vi "Set Front Panel Visibility.vi"(6 "Set Value":bool, 9 "Elapsed Time":dbl, 10 "Current Tab":T1(ring), 11 "output cluster":T2) -> (3 "New Tab":T1(ring))   [LabVIEW 2016]
uses:
  Controls/Cal Refs.ctl
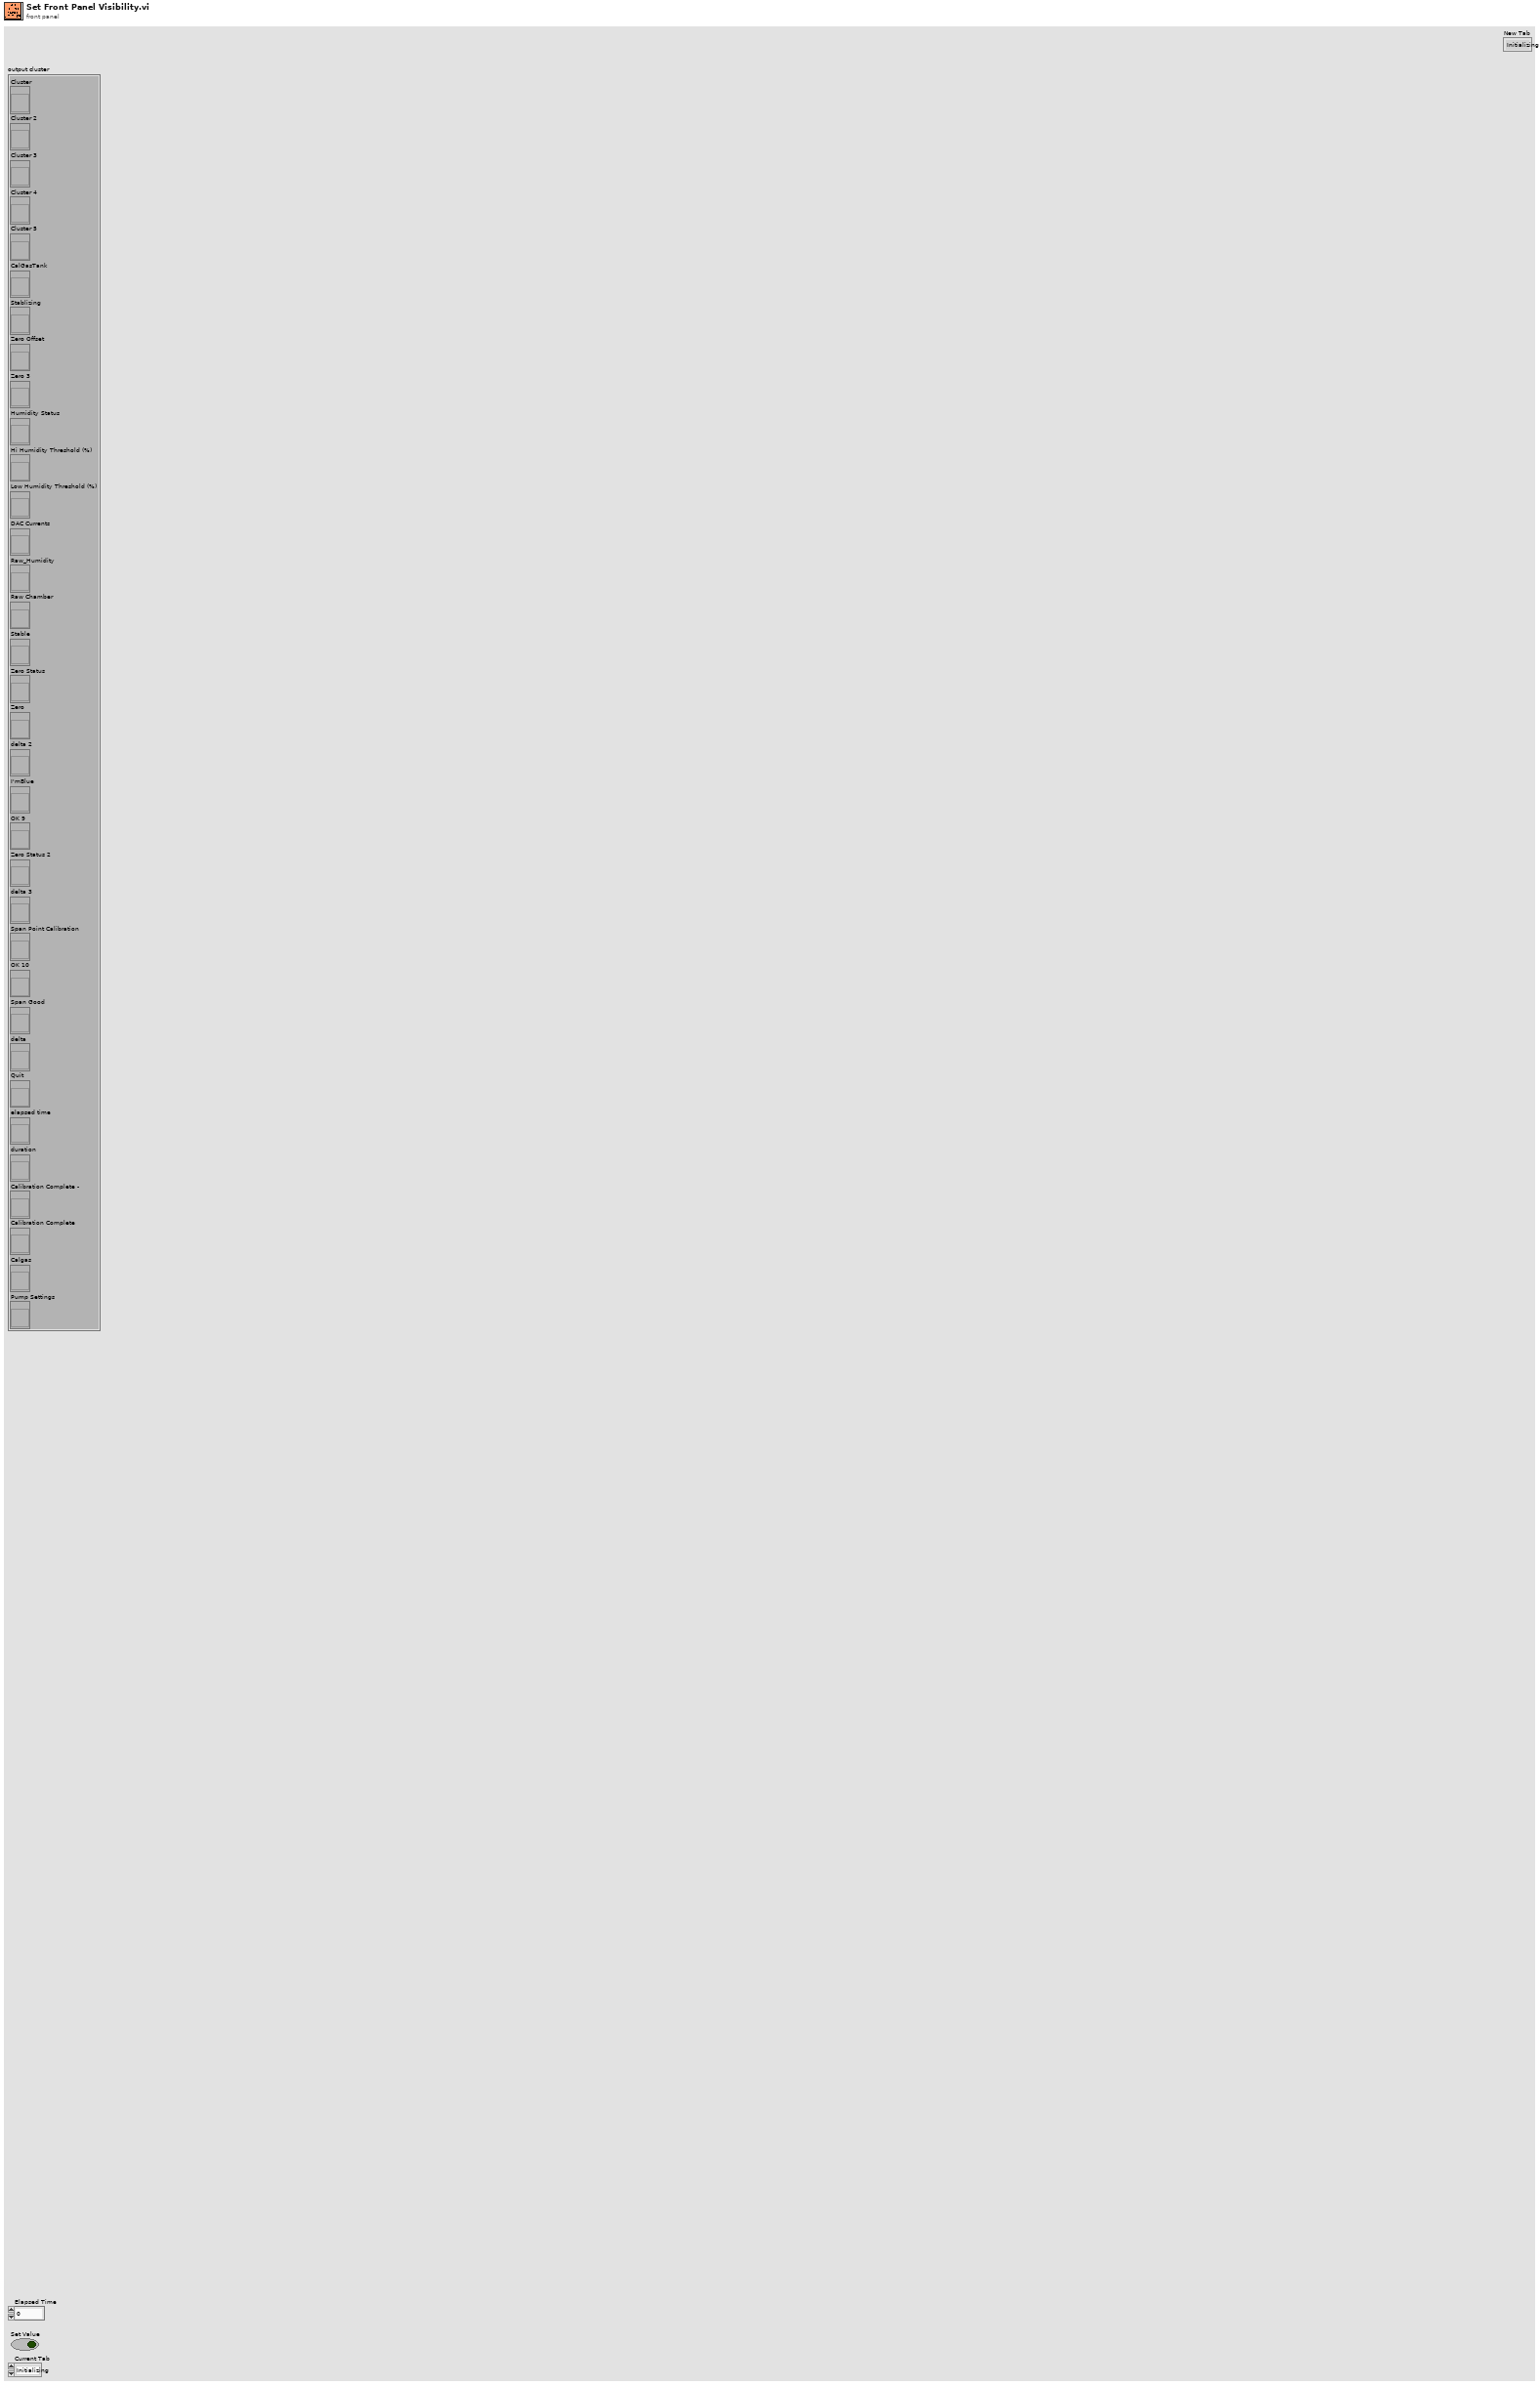
[diagram p1: front panel]
types:
  T1 = enum32{"Initializing", "Enter CO2 Value", "Enter Calibration Code", "Reading Calibration Data", "Stablizing", "Calculating Target Voltages", "Setting Zero Point", "Setting High Point", "Setting Span Point", "Calculating Gain & Offset", "Storing Calibration Coefficients", "Calibration Complete"}
  T2 = typedef "Cal Refs.ctl" = cluster{"Cluster":refnum<vi>, "Cluster 2":refnum<vi>, "Cluster 3":refnum<vi>, "Cluster 4":refnum<vi>, "Cluster 5":refnum<vi>, "CalGasTank":refnum<vi>, "Stablizing":refnum<vi>, "Zero Offset":refnum<vi>, "Zero 3":refnum<vi>, "Humidity Status":refnum<vi>, "Hi Humidity Threshold (%)":refnum<vi>, "Low Humidity Threshold (%)":refnum<vi>, "DAC Currents":refnum<vi>, "Raw_Humidity":refnum<vi>, "Raw Chamber":refnum<vi>, "Stable":refnum<vi>, "Zero Status":refnum<vi>, "Zero":refnum<vi>, "delta 2":refnum<vi>, "I'mBlue":refnum<vi>, "OK 9":refnum<vi>, "Zero Status 2":refnum<vi>, "delta 3":refnum<vi>, "Span Point Calibration":refnum<vi>, "OK 10":refnum<vi>, "Span Good":refnum<vi>, "delta":refnum<vi>, "Quit":refnum<vi>, "elapsed time":refnum<vi>, "duration":refnum<vi>, "Calibration Complete -":refnum<vi>, "Calibration Complete":refnum<vi>, "Calgas":refnum<vi>, "Pump Settings":refnum<vi>}
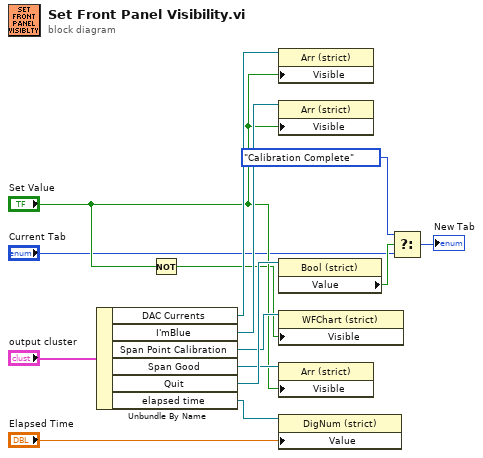
[diagram p0: block diagram]
diagram:
  n1 = Unbundle By Name("output cluster") -> ("DAC Currents"=w7:refnum<vi>, "I'mBlue"=w8:refnum<vi>, "Span Point Calibration"=w9:refnum<vi>, "Span Good"=w10:refnum<vi>, "Quit"=w11:refnum<vi>, "elapsed time"=w13:refnum<vi>)
  n2 = Not(x="Set Value") -> (.not. x?=w3:bool)
  n3 = property on="Property Node" class="Arr (strict)"(reference=w7, "Visible"="Set Value") -> ()  [unwired: 1 in, 2 out]
  n4 = property on="Property Node" class="Arr (strict)"(reference=w8, "Visible"="Set Value") -> ()  [unwired: 1 in, 2 out]
  n5 = property class="Bool (strict)"(reference=w11) -> ("Value"=w12:bool)  [unwired: 1 in, 2 out]
  n6 = property on="Property Node" class="WFChart (strict)"(reference=w9, "Visible"=w3) -> ()  [unwired: 1 in, 2 out]
  n7 = property on="Property Node" class="Arr (strict)"(reference=w10, "Visible"="Set Value") -> ()  [unwired: 1 in, 2 out]
  n8 = property class="DigNum (strict)"(reference=w13, "Value"="Elapsed Time") -> ()  [unwired: 1 in, 2 out]
  n9 = Select(t=T1."Calibration Complete" ("CalStatusTab"), s=w12, f="Current Tab") -> (s? t:f=→"New Tab":T1)
